vi "DataType to Register Size.vi"(11 "DataType":T1) -> (2 "bits":i32, 3 "Registers":i32)   [LabVIEW 2021, in "Modbus Master Shared.lvlib"]
uses:
  Shared/Modbus Master Shared.lvlib
  Shared/Controls/Data Model/DataType.ctl
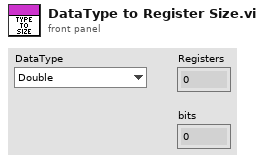
[diagram p1: front panel]
types:
  T1 = typedef "Modbus Master Shared.lvlib/DataType.ctl" = enum16{"Double", "Single", "I64", "I32", "I16", "I8", "U64", "U32", "U16", "U8", "Boolean"}
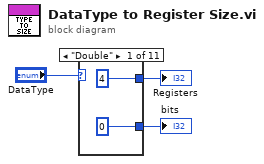
[diagram p0: block diagram]
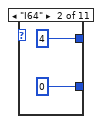
[diagram p2: hidden frame]
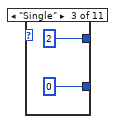
[diagram p3: hidden frame]
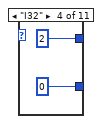
[diagram p4: hidden frame]
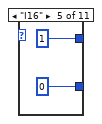
[diagram p5: hidden frame]
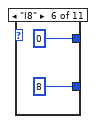
[diagram p6: hidden frame]
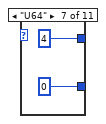
[diagram p7: hidden frame]
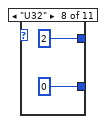
[diagram p8: hidden frame]
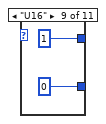
[diagram p9: hidden frame]
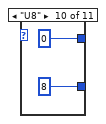
[diagram p10: hidden frame]
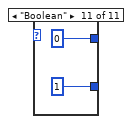
[diagram p11: hidden frame]
diagram:
  n1 = case shown="\"Double\"" "DataType" {
    tunnel: [4 4 2 2 1 0 4 2 1 0 0] -> w2
    tunnel: [0 0 0 0 0 8 0 0 0 8 1] -> w3
    frame "Double" {
    }
    frame "I64" {
    }
    frame "Single" {
    }
    frame "I32" {
    }
    frame "I16" {
    }
    frame "I8" {
    }
    frame "U64" {
    }
    frame "U32" {
    }
    frame "U16" {
    }
    frame "U8" {
    }
    frame "Boolean" {
    }
  }
  "bits" <- w3
  "Registers" <- w2
